vi "WFM MNGR Add ET Waveform to PropertyObject.vi"(8 "error in (no error)":errorcluster, 10 "ET Waveform":T1, 11 "WFM MNGR in":refnum<class "QPA MSMT Waveform Manager.lvclass">) -> (0 "error out":errorcluster, 3 "WFM MNGR out":refnum<class "QPA MSMT Waveform Manager.lvclass">)   [LabVIEW 2016, in "QPA MSMT Waveform Manager.lvclass"]
uses:
  QPA MSMT Waveform Manager.lvclass
  Controls/ET Waveform.ctl
  QPA MSMT Waveform Manager.lvclass/QPA MSMT Waveform Manager.ctl
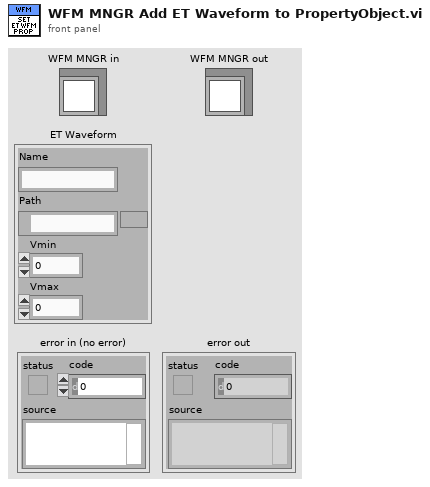
[diagram p1: front panel]
types:
  T1 = typedef "QPA MSMT Waveform Manager.lvclass/ET Waveform.ctl" = cluster{"Name":string, "Path":path, "Vmin":dbl, "Vmax":dbl}
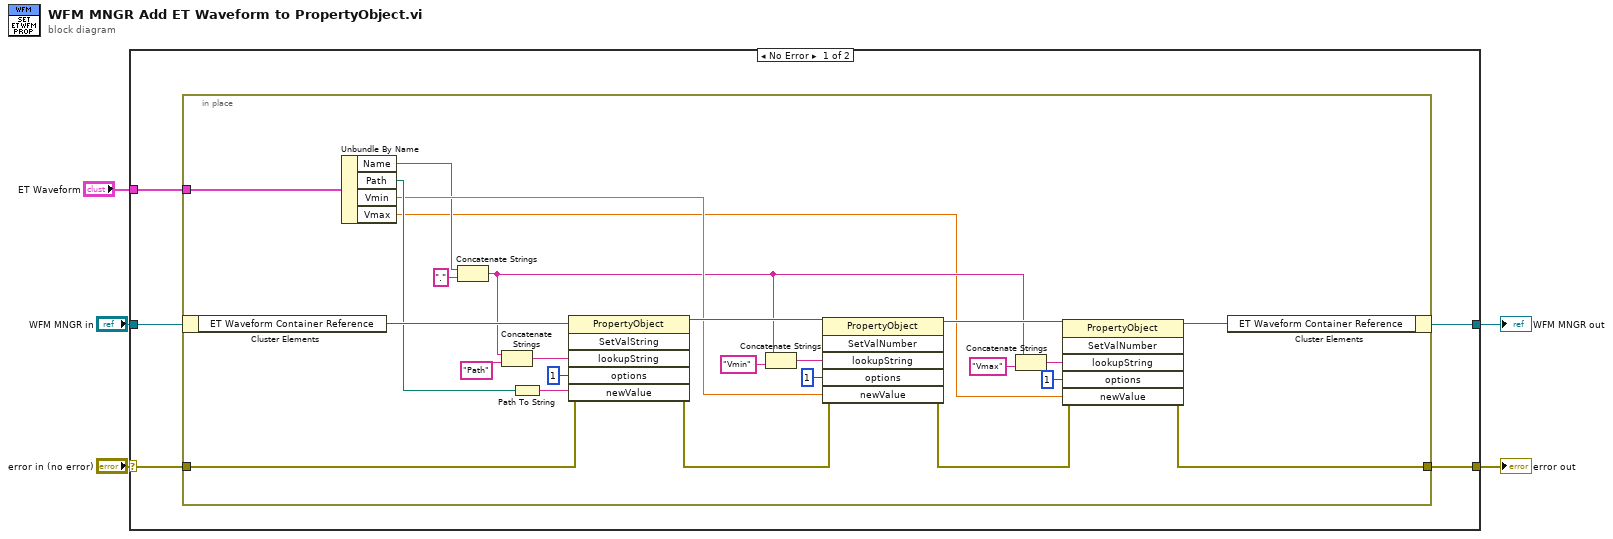
[diagram p0: block diagram]
diagram:
  n1 = case shown="No Error" "error in (no error)" {
    selector: "error in (no error)" -> [w8 w37]
    tunnel: [w6 w37] -> w4
    tunnel: [w9 w36] -> w2
    tunnel: "WFM MNGR in" -> [w10 w36]
    tunnel: "ET Waveform" -> [w7 _]
    frame No Error {
      n2 = in-place {
        in-place-border: w8 -> [w33]
        in-place-border: w7 -> [w35]
        in-place-border: [w17] -> w6
        n3 = in-place-cluster #1(w10) -> ("ET Waveform Container Reference"=w34:refnum<k7>)
        n4 = Unbundle By Name(w35) -> ("Name"=w23:string, "Path"=w29:path, "Vmin"=w24:dbl, "Vmax"=w11:dbl)
        n5 = Concatenate Strings(w23, "." ("string")) -> (w15:string)
        n6 = Concatenate Strings(w15, "Path" ("string")) -> (w28:string)
        n7 = Path To String(path=w29) -> (string=w30:string)
        n8 = invoke class="PropertyObject" method="SetValString"(reference=w34, error in=w33, "lookupString"=w28, "options"=1, "newValue"=w30) -> (reference out=w26:refnum<k7>, error out=w25:errorcluster)  [unwired: 1 in, 4 out]
        n9 = Concatenate Strings(w15, "Vmin" ("string")) -> (w22:string)
        n10 = invoke class="PropertyObject" method="SetValNumber"(reference=w26, error in=w25, "lookupString"=w22, "options"=1, "newValue"=w24) -> (reference out=w20:refnum<k7>, error out=w18:errorcluster)  [unwired: 1 in, 4 out]
        n11 = Concatenate Strings(w15, "Vmax" ("string")) -> (w16:string)
        n12 = invoke class="PropertyObject" method="SetValNumber"(reference=w20, error in=w18, "lookupString"=w16, "options"=1, "newValue"=w11) -> (reference out=w19:refnum<k7>, error out=w17:errorcluster)  [unwired: 1 in, 4 out]
        n13 = in-place-cluster #1("ET Waveform Container Reference"=w19) -> (w9:refnum<class "QPA MSMT Waveform Manager.lvclass">)
      }
    }
    frame Error {
    }
  }
  "error out" <- w4
  "WFM MNGR out" <- w2
